vi "Set Averaging ILD1420.vi"(0 "COM port":refnum<visa-resource-name>, 7 "Averaging mode":string(combo)="NONE", 9 "Averaging depth":u16=9) -> (15 "Error out":errorcluster)   [LabVIEW 2015]
uses:
  Ctls/Cmd_ILD1420.ctl
panel:
  # "PN 11/08/2016"
  # "-- MOVING: Moving averaging value (averaging depth 2, 4, 8, 16, 32, 64 and 128 possible)\n-- RECURSIVE: Recursive averaging value (averaging depth 1 up to 32768 possible)\n-- MEDIAN: Median (averaging depth 3, 5, 7 and 9 possible)"
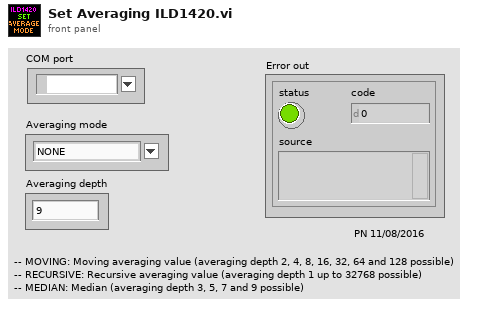
[diagram p1: front panel]
types:
  T1 = typedef "Cmd_ILD1420.ctl" = string
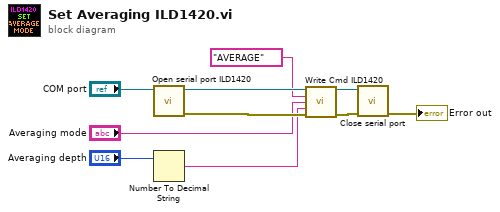
[diagram p0: block diagram]
diagram:
  n1 = call "Open serial port ILD1420.vi"("VISA resource name"="COM port") -> ("Error out"=w9:errorcluster, "VISA resource name out"=w8:refnum<visa-resource-name>)  [unwired: 9 in]
  n2 = Number To Decimal String(number="Averaging depth") -> (decimal integer string=w1:string)  [unwired: 1 in]
  n3 = call "Write Cmd ILD1420.vi"("COM port"=w8, "Cmd"=T1 "AVERAGE", "Param1"="Averaging mode", "Param2"=w1, "Error in"=w9) -> ("COM port out"=w7:refnum<visa-resource-name>, "Error out"=w6:errorcluster)  [unwired: 9 in]
  n4 = call "Close serial port.vi"("Error in"=w6, "VISA resource name"=w7) -> ("Error out"=→"Error out":errorcluster)  [unwired: 9 in]
